vi "Tx Section Page.vi"(8 "error in (no error)":errorcluster, 11 "Node Ptr":T1 format="%.0x") -> (0 "error out":errorcluster)   [LabVIEW 2019, in "UDP-Custom-Device System Explorer.lvlib"]
uses:
  UDP-Custom-Device System Explorer.lvlib
  <vilib>/NI VeriStand/Custom Device API/Custom Device Item Ref.ctl
  <vilib>/NI VeriStand/Custom Device API/Custom Device API.lvlib
  Property Accessors/Shared Section Accessors.lvlib
panel:
  in  "Tx Packets":i32[](listbox)
  in  "SHDocVw.IWebBrowser":refnum<k7>(container)
  in  "General Header":cluster{"Section Name":string}={"Section Name"="Configured Packets"}
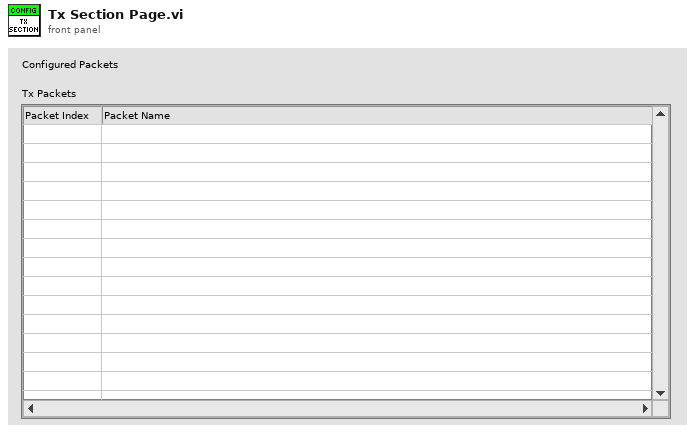
[diagram p1: front panel]
types:
  T1 = typedef "Custom Device API.lvlib/Custom Device Item Ref.ctl" = u64
  T2 = typedef "Custom Device API.lvlib/Custom Device Commands.ctl" = enum16{"Default", "Item renamed", "Shutdown", "Dynamic button pressed"}
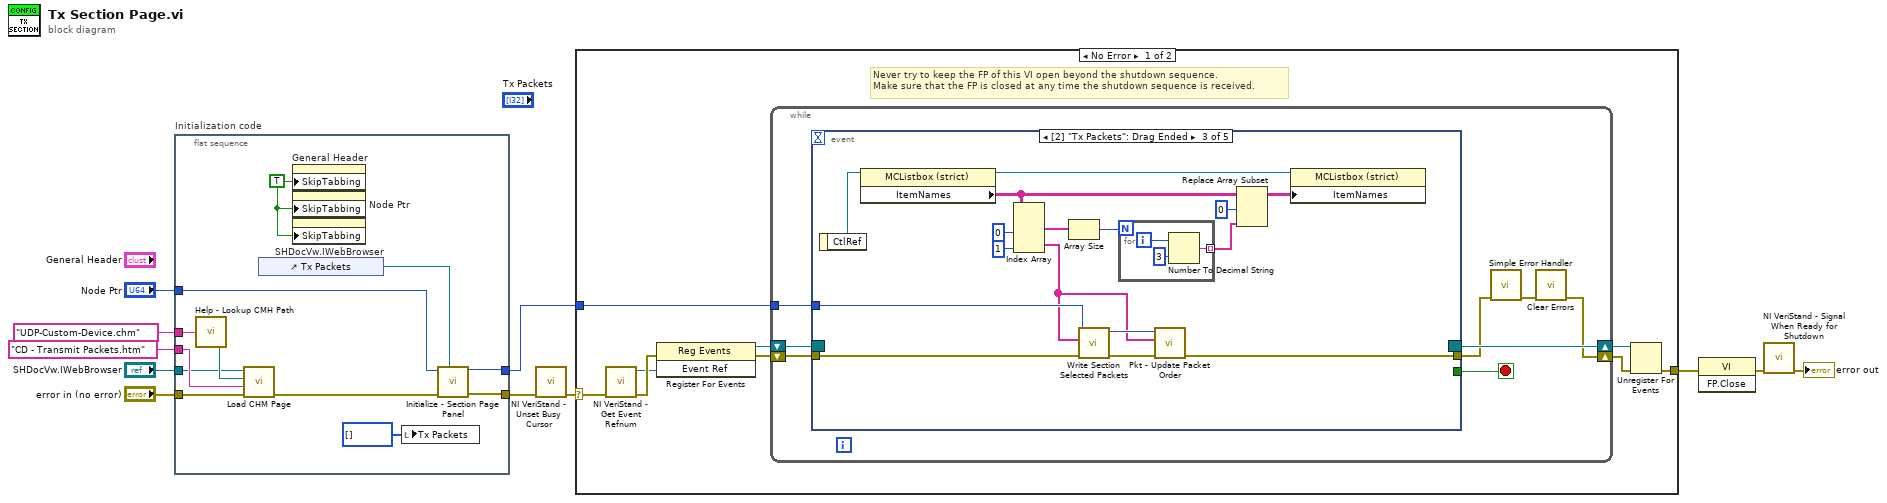
[diagram p0: block diagram]
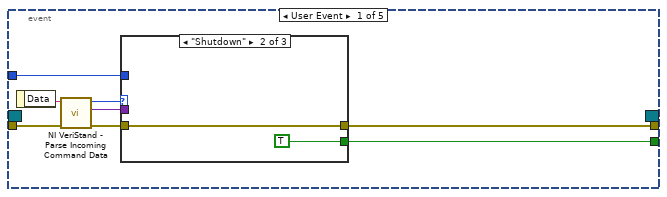
[diagram p2: hidden frame]
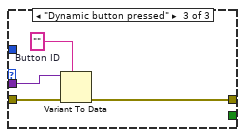
[diagram p4: hidden frame]
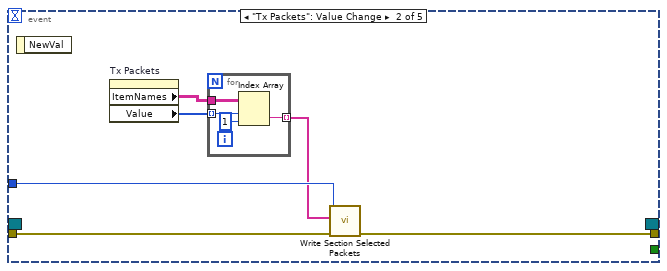
[diagram p5: hidden frame]
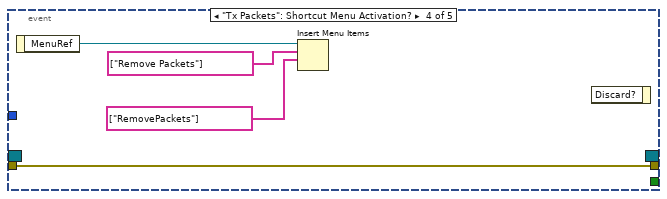
[diagram p6: hidden frame]
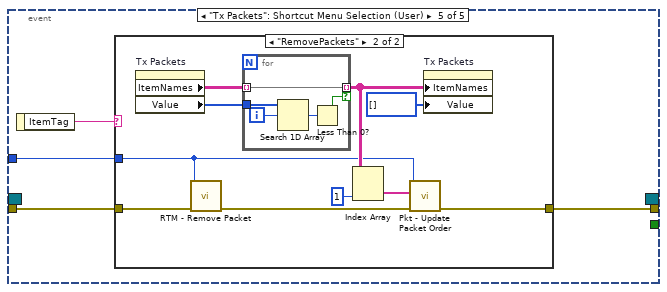
[diagram p7: hidden frame]
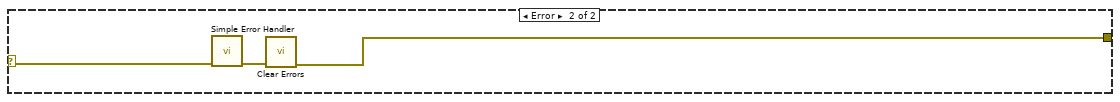
[diagram p9: hidden frame]
diagram:
  n1 = flat-sequence "Initialization code" {
    tunnel: "error in (no error)" -> [w19]
    tunnel: "Node Ptr" -> [w21]
    tunnel: [w23] -> w7
    tunnel: [w22] -> w4
    tunnel: "SHDocVw.IWebBrowser" -> [w16]
    tunnel: "CD - Transmit Packets.htm" ("CD_CHM_Section") -> [w17]
    tunnel: "UDP-Custom-Device.chm" ("CD_CHM_FileName") -> [w18]
    frame #0 {
      w12 = TRUE ("Skip When Tabbing")
      n2 = call "Help - Lookup CMH Path.vi"("Main CMH File"=w18) -> ("Compiled CMH Path"=w20:path)
      n3 = call <vilib>:"Load CHM Page.vi"("error in (no error)"=w19, "HTML File"=w17, "Compiled CHM Path"=w20, "Web Browser Reference"=w16) -> ("error out"=w15:errorcluster)  [unwired: 7 in]
      n4 = control-ref of="Tx Packets"() -> (w13:refnum<vi>)
      n5 = property on="General Header" class="Clust (strict)"("SkipTabbing"=w12) -> ()  [unwired: 2 in, 2 out]
      n6 = property on="Node Ptr" class="DigNum (strict)"("SkipTabbing"=w12) -> ()  [unwired: 2 in, 2 out]
      n7 = property on="SHDocVw.IWebBrowser" class="AXCont"("SkipTabbing"=w12) -> ()  [unwired: 2 in, 2 out]
      n8 = local write "Tx Packets"(i32[] [] ("Tx Packets")) -> ()
      n9 = call "Initialize - Section Page Panel.vi"("Packets Listbox"=w13, "error in (no error)"=w15, "Item Ref in"=w21) -> ("error out"=w23:errorcluster, "Item Ref out"=w22:T1)  [unwired: 7 in]
    }
  }
  n10 = call <vilib>:"NI VeriStand - Unset Busy Cursor.vi"("error in (no error)"=w7) -> ("error out"=w6:errorcluster)  [unwired: 10 out]
  n11 = case shown="No Error" w6 {
    selector: w6 -> [w24 w111]
    tunnel: [w29 w109] -> w11
    tunnel: w4 -> [w25 _]
    frame No Error {
      # "Never try to keep the FP of this VI open beyond the shutdown sequence.\nMake sure that the FP is closed at any time the shutdown sequence is received."
      n12 = call <vilib>:"NI VeriStand - Get Event Refnum.vi"("error in (no error)"=w24) -> ("error out"=w32:errorcluster, "Event Ref"=w28:refnum<user-event>)  [unwired: 9 out]
      n13 = register-events(error in=w32, w28) -> (reference out=w26:refnum<event-registration>, error out=w27:errorcluster)  [unwired: 1 in]
      n14 = while {
        tunnel: w25 -> [w36]
        shift-right: [w33] -> w30
        shift-left: w27 -> [w39]
        shift-right: [w40] -> w31
        shift-left: w26 -> [w38]
        stop <- w37 stop-if-true
        n15 = event shown="[2] \"Tx Packets\": Drag Ended" {
          selector: w38 -> [_ _ _ _ _]
          dyn-events: [_ _ _ _ _] -> w40
          timeout: _ -> [_ _ _ _ _]
          tunnel: w39 -> [w48 w58 w72 w85 w90]
          tunnel: [w44 _ _ _ _] -> w37
          tunnel: [w43 w57 w74 w85 w89] -> w35
          tunnel: w36 -> [w42 w59 w73 _ w91]
          event User Event {
            n16 = event-data() -> ("Data"=w47:string)  [unwired: 1 out]
            n17 = call <vilib>:"NI VeriStand - Parse Incoming Command Data.vi"("error in (no error)"=w48, "Incoming data"=w47) -> ("error out"=w46:errorcluster, "Outgoing data"=w41:variant, "Action"=w45:T2)  [unwired: 7 out]
            n18 = case shown="\"Shutdown\"" w45 {
              tunnel: w46 -> [w49 w50 w55]
              tunnel: [_ TRUE _] -> w44
              tunnel: [w49 w50 w52] -> w43
              tunnel: w42 -> [_ _ _]
              tunnel: w41 -> [_ _ w54]
              frame "Default", Default {
              }
              frame "Shutdown" {
              }
              frame "Dynamic button pressed" {
                w53 = ""  # Button ID
                n19 = Variant To Data(error in=w55, type=w53, Variant=w54) -> (error out=w52:errorcluster)  [unwired: 1 out]
              }
            }
          }
          event "Tx Packets": Value Change {
            n20 = event-data() -> ()  [unwired: 2 out]
            n21 = property on="Tx Packets" class="MCListbox (strict)"() -> ("ItemNames"=w61:string[][], "Value"=w60:i32[])  [unwired: 2 in, 2 out]
            n22 = for {
              tunnel: w61 -> [w65]
              tunnel: [w64] -> w56 mode=indexing
              tunnel: w60 -> [w63] mode=indexing
              n23 = Index Array(array=w65, index (row)=w63, index (col)=1 ("disabled index (row)")) -> (element=w64:string)
            }
            n24 = call "Write Section Selected Packets.vi"("error in (no error)"=w58, "Selected Packets"=w56, "Node Ptr"=w59) -> ("error out"=w57:errorcluster)  [unwired: 7 in, 1 out]
          }
          event "Tx Packets": Drag Ended {
            n25 = event-data() -> ("CtlRef"=w69:refnum<vi>)  [unwired: 1 out]
            n26 = property class="MCListbox (strict)"(reference=w69) -> (reference out=w68:refnum<vi>, "ItemNames"=w75:string[][])  [unwired: 1 in, 1 out]
            n27 = Index Array(array=w75, index (col) #1=0 ("disabled index (col)"), index (col) #2=1 ("index (col)")) -> (element #1=w79:string[], element #2=w66:string[])  [unwired: 2 in]
            n28 = Array Size(array=w79) -> (size(s)=w78:i32)
            n29 = call "Write Section Selected Packets.vi"("error in (no error)"=w72, "Selected Packets"=w66, "Node Ptr"=w73) -> ("error out"=w71:errorcluster, "Node Ptr out"=w70:T1)  [unwired: 7 in]
            n30 = for {
              N: w78 -> [_]
              tunnel: [w82] -> w76 mode=indexing
              i -> [w84]
              n31 = Number To Decimal String(number=w84, width (-)=i16 3) -> (decimal integer string=w82:string)
            }
            n32 = call "Pkt - Update Packet Order.vi"("error in (no error)"=w71, "Channel Names"=w66, "Node Ptr"=w70) -> ("error out"=w74:errorcluster)  [unwired: 7 in, 1 out]
            n33 = Replace Array Subset(array=w75, new element=w76, index (col)=0 ("disabled index (col)")) -> (w81:string[][])  [unwired: 1 in]
            n34 = property class="MCListbox (strict)"(reference=w68, "ItemNames"=w81) -> ()  [unwired: 1 in, 2 out]
          }
          event "Tx Packets": Shortcut Menu Activation? {
            n35 = event-data() -> ("MenuRef"=w86:refnum<k9>)  [unwired: 1 out]
            n36 = Insert Menu Items(7:string[] ["RemovePackets"] ("item names"), 8:string[] ["Remove Packets"] ("item names"), 9:w86) -> ()  [unwired: 3 in, 3 out]
            n37 = event-data() -> ()  [unwired: 2 in, 1 out]
          }
          event "Tx Packets": Shortcut Menu Selection (User) {
            n38 = event-data() -> ("ItemTag"=w92:string)  [unwired: 1 out]
            n39 = case shown="\"RemovePackets\"" w92 {
              tunnel: w91 -> [_ w95]
              tunnel: w90 -> [w93 w103]
              tunnel: [w93 w96] -> w89
              frame Default {
              }
              frame "RemovePackets" {
                n40 = property on="Tx Packets" class="MCListbox (strict)"() -> ("ItemNames"=w101:string[][], "Value"=w102:i32[])  [unwired: 2 in, 2 out]
                n41 = call "RTM - Remove Packet.vi"("error in (no error)"=w103, "Node Ptr"=w95) -> ("error out"=w97:errorcluster)  [unwired: 9 in]
                n42 = for {
                  tunnel: w102 -> [w106]
                  tunnel: [w108] -> w98 mode=indexing if=w104
                  tunnel: w101 -> [w108] mode=indexing
                  i -> [w105]
                  n43 = Search 1D Array(1D array=w106, element=w105) -> (index of element=w107:i32)  [unwired: 1 in]
                  n44 = Less Than 0?(x=w107) -> (x < 0?=w104:bool)
                }
                n45 = Index Array(array=w98, index (col)=1 ("disabled index (col)")) -> (element=w94:string[])  [unwired: 1 in]
                n46 = call "Pkt - Update Packet Order.vi"("error in (no error)"=w97, "Channel Names"=w94, "Node Ptr"=w95) -> ("error out"=w96:errorcluster)  [unwired: 7 in, 1 out]
                n47 = property on="Tx Packets" class="MCListbox (strict)"("ItemNames"=w98, "Value"=i32[] [] ("Tx Packets")) -> ()  [unwired: 2 in, 2 out]
              }
            }
          }
        }
        n48 = call <vilib>:"Simple Error Handler.vi"("error in (no error)"=w35) -> ("error out"=w34:errorcluster)  [unwired: 1 in, 7 out]
        n49 = call <vilib>:"Clear Errors.vi"("error in (no error)"=w34) -> ("error out"=w33:errorcluster)  [unwired: 1 in, 5 out]
      }
      n50 = Unregister For Events(event registration refnum=w31, error in=w30) -> (error out=w29:errorcluster)
    }
    frame Error {
      n51 = call <vilib>:"Simple Error Handler.vi"("error in (no error)"=w111) -> ("error out"=w110:errorcluster)  [unwired: 1 in, 7 out]
      n52 = call <vilib>:"Clear Errors.vi"("error in (no error)"=w110) -> ("error out"=w109:errorcluster)  [unwired: 1 in, 5 out]
    }
  }
  n53 = invoke class="VI" method="FP.Close"(error in=w11) -> (error out=w10:errorcluster)  [unwired: 2 in, 2 out]
  n54 = call <vilib>:"NI VeriStand - Signal When Ready for Shutdown.vi"("error in (no error)"=w10) -> ("error out"=→"error out":errorcluster)  [unwired: 10 out]
